vi "High Speed Reading.vi"() -> ()   [LabVIEW 2018]
uses:
  TwinCAT ADS Class/VIs/Build G Object From Btye Stream.vi
  TwinCAT ADS Class/TwinCAT ADS.lvclass
panel:
  out "Elapsed Time /s":dbl=0.00098230000003241 format="%^#_6e"
  out "Value":variant
  in  "Stop":bool
  # "PLC Cycle Time  was 1ms"
  # "Example PLC Source Code is available at:\nhttps://github.com/fisothemes/LabVIEW-TwinCAT-ADS/tree/master/src/PLC"
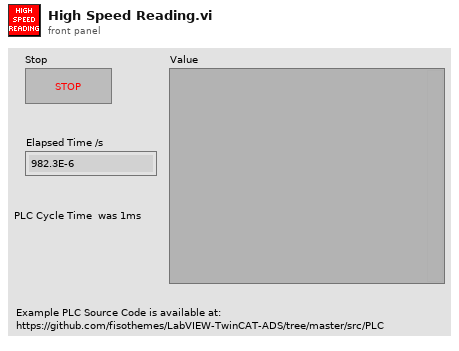
[diagram p1: front panel]
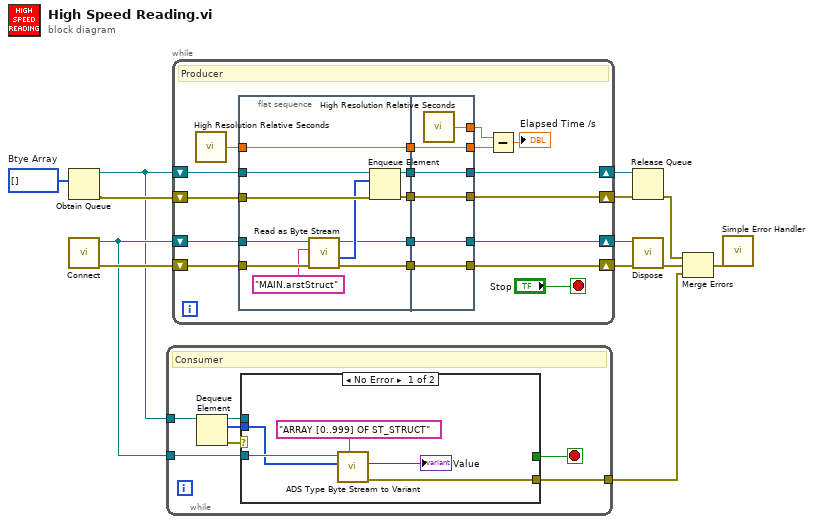
[diagram p0: block diagram]
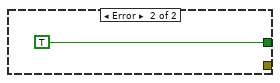
[diagram p2: hidden frame]
diagram:
  w11 = u8[] []  # Btye Array
  n1 = Obtain Queue(element data type=w11) -> (queue out=w9:refnum<queue>, error out=w13:errorcluster)  [unwired: 4 in, 1 out]
  n2 = call "Connect.vi"() -> ("error out"=w12:errorcluster, "TwinCAT ADS out"=w10:refnum<class "TwinCAT ADS.lvclass">)  [unwired: 10 in]
  n3 = while {
    tunnel: w10 -> [w17]
    tunnel: w9 -> [w20]
    tunnel: [w14] -> w1
    stop <- w15 stop-if-true
    # "Consumer"
    n4 = Dequeue Element(queue=w20) -> (queue out=w16:refnum<queue>, element=w18:u8[], error out=w19:errorcluster)  [unwired: 2 in, 1 out]
    n5 = case shown="No Error" w19 {
      tunnel: w18 -> [w23 _]
      tunnel: w17 -> [w25 _]
      tunnel: [_ TRUE ("status")] -> w15
      tunnel: w16 -> [_ _]
      tunnel: [w21 _] -> w14
      frame No Error {
        n6 = call "ADS Type Byte Stream to Variant.vi"("Type Name"="ARRAY [0..999] OF ST_STRUCT", "Byte Stream"=w23, "TwinCAT ADS in"=w25) -> ("error out"=w21:errorcluster, "Value"=→"Value":variant)  [unwired: 6 in, 1 out]
      }
      frame Error {
      }
    }
  }
  n7 = while {
    shift-right: [w40] -> w8
    shift-left: w10 -> [w43]
    shift-right: [w41] -> w5
    shift-left: w9 -> [w44]
    shift-right: [w38] -> w7
    shift-left: w12 -> [w37]
    shift-right: [w39] -> w6
    shift-left: w13 -> [w42]
    stop <- "Stop" stop-if-true
    # "Producer"
    n8 = call <vilib>:"High Resolution Relative Seconds.vi"() -> ("relative seconds"=w35:dbl)
    n9 = flat-sequence {
      tunnel: w44 -> [w55]
      tunnel: w43 -> [w54]
      tunnel: w42 -> [w53]
      tunnel: w37 -> [w47]
      tunnel: w35 -> [w45]
      tunnel: [w51] -> w34
      tunnel: [w50] -> w33
      tunnel: [w49] -> w32
      tunnel: [w48] -> w31
      tunnel: [w45] -> w30
      tunnel: [w57] -> w28
      tunnel: [w58] -> w38
      tunnel: [w59] -> w39
      tunnel: [w60] -> w40
      tunnel: [w61] -> w41
      tunnel: w34 -> [w61]
      tunnel: w33 -> [w60]
      tunnel: w32 -> [w59]
      tunnel: w31 -> [w58]
      tunnel: w30 -> [w57]
      tunnel: [w56] -> w29
      frame #0 {
        n10 = call "Read as Byte Stream.vi"("error in (no error)"=w47, "Symbol Name"="MAIN.arstStruct", "TwinCAT ADS in"=w54) -> ("error out"=w48:errorcluster, "Byte Stream out"=w52:u8[], "TwinCAT ADS out"=w50:refnum<class "TwinCAT ADS.lvclass">)  [unwired: 6 in]
        n11 = Enqueue Element(queue=w55, element=w52, error in (no error)=w53) -> (queue out=w51:refnum<queue>, error out=w49:errorcluster)  [unwired: 1 in, 1 out]
      }
      frame #1 {
        n12 = call <vilib>:"High Resolution Relative Seconds.vi"() -> ("relative seconds"=w56:dbl)
      }
    }
    n13 = Subtract(x=w29, y=w28) -> (x-y=→"Elapsed Time /s":dbl)
  }
  n14 = Release Queue(queue=w5, error in (no error)=w6) -> (error out=w4:errorcluster)  [unwired: 1 in, 2 out]
  n15 = call "Dispose.vi"("error in (no error)"=w7, "TwinCAT ADS in"=w8) -> ("error out"=w3:errorcluster)  [unwired: 9 in]
  n16 = Merge Errors(w4, w3, w1) -> (w2:errorcluster)
  n17 = call <vilib>:"Simple Error Handler.vi"("error in (no error)"=w2) -> ()  [unwired: 4 in, 5 out]
